vi "DAQAI.vi"(2 "rate":dbl=1000.0, 3 "number of samples":i32=1000, 4 "timeout (s)":dbl=10.0 format="%0.2f", 5 "error in":errorcluster, 7 "stop (F)":bool, 10 "device name":tag="Dev1") -> (14 "task out":refnum<k21>, 15 "data":dynamicdata(graph), 18 "stopped":bool, 19 "error out":errorcluster)   [LabVIEW 2018]
doc: "Creates, edits, and runs tasks using NI-DAQmx. Refer to the NI-DAQmx Readme for a complete listing of devices NI-DAQmx supports.\n\nWhen you place this Express VI on the block diagram, the DAQ Assistant launches to create a new task. After you create a task, you can double-click the DAQ Assistant Express VI to edit that task. For continuous measurement or generation, place a while loop around the DAQ Assistant Express VI."
uses:
  <vilib>/DAQmx/read.llb/DAQmx Read.vi
  <vilib>/DAQmx/read.llb/DAQmx Read (Analog 1D Wfm NChan NSamp).vi
  <vilib>/DAQmx/create/channels.llb/DAQmx Create Channel (TEDS-AI-Voltage-Basic).vi
  <vilib>/DAQmx/create/channels.llb/DAQmx Create Channel (AI-Voltage-Basic).vi
  <vilib>/DAQmx/configure/timing.llb/DAQmx Timing (Sample Clock).vi
  <vilib>/DAQmx/miscellaneous.llb/DAQmx Fill In Error Info.vi
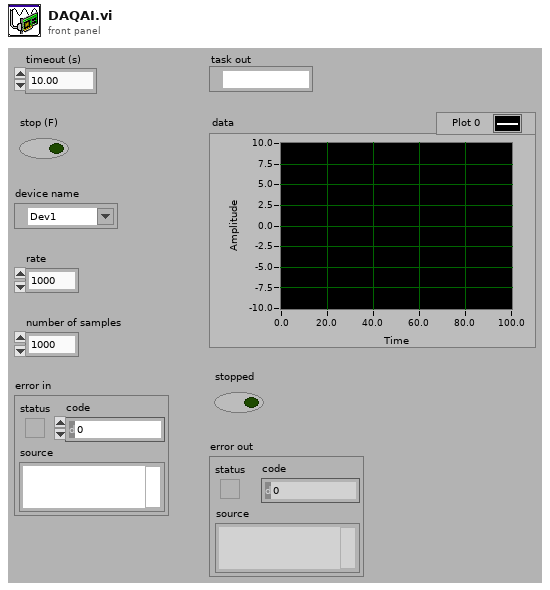
[diagram p1: front panel]
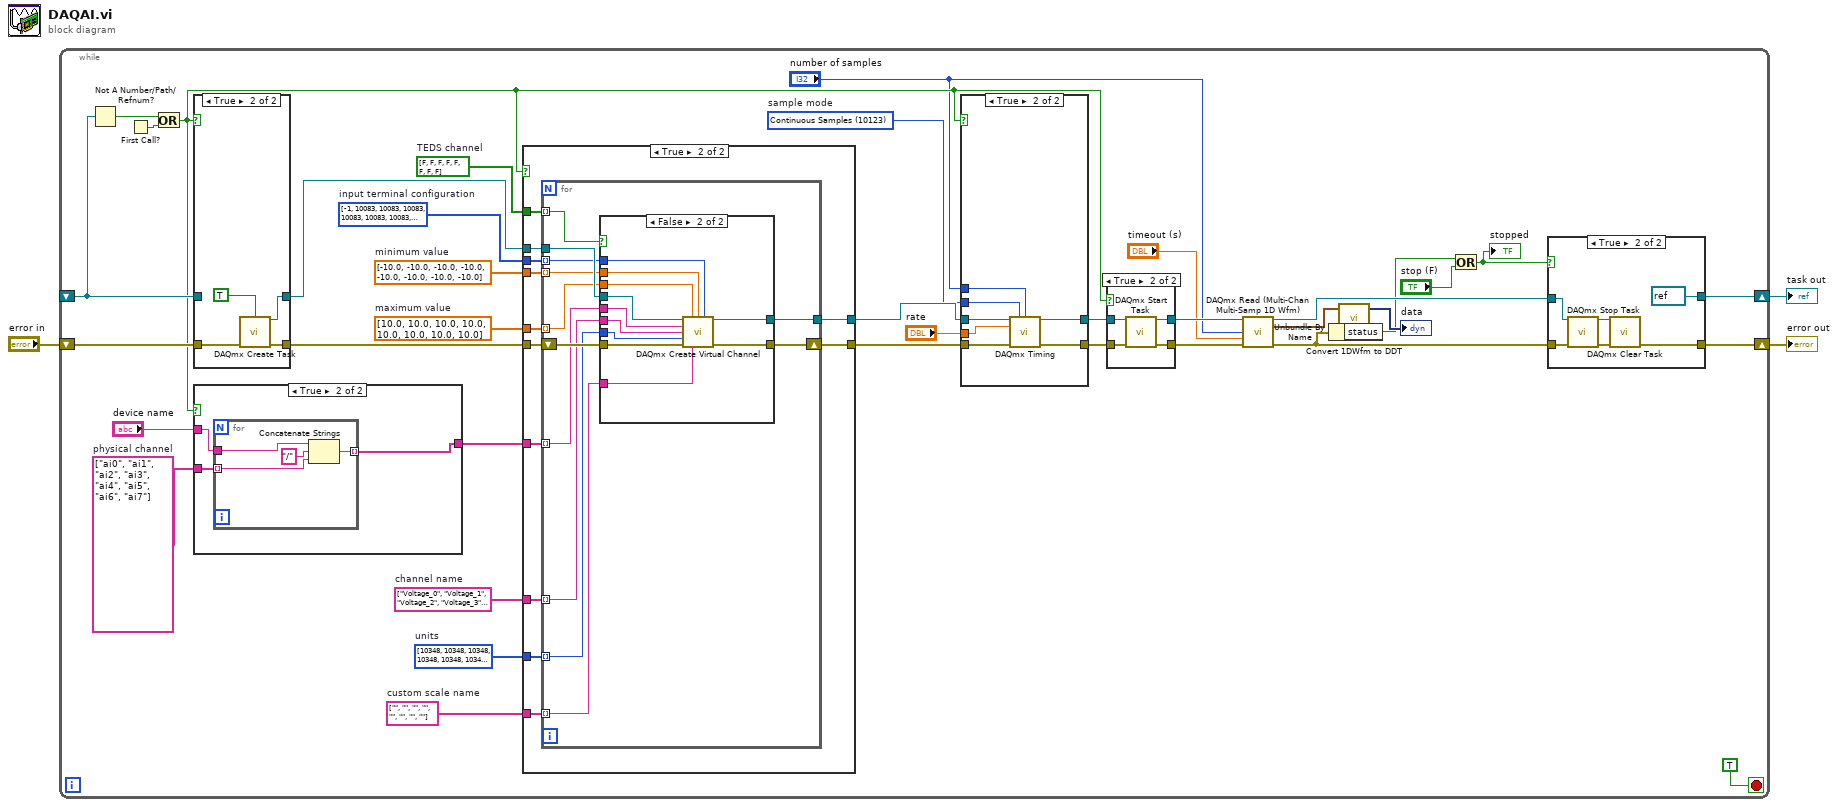
[diagram p0: block diagram]
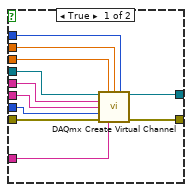
[diagram p6: hidden frame]
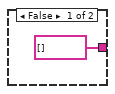
[diagram p7: hidden frame]
diagram:
  n1 = while {
    shift-right: [w10] -> w1
    shift-left: _ -> [w37]
    shift-right: [w8] -> w2
    shift-left: "error in" -> [w38]
    stop <- TRUE stop-if-true
    w20 = 10123 items=["Finite Samples"=10178, "Continuous Samples"=10123, "Hardware Timed Single Point"=12522]  # sample mode
    w24 = bool[] [FALSE, FALSE, FALSE, FALSE, FALSE, FALSE, FALSE, FALSE]  # TEDS channel
    w25 = string[] ["", "", "", "", "", "", "", ""]  # custom scale name
    w26 = i32[] [10348, 10348, 10348, 10348, 10348, 10348, 10348, 10348] items=["Volts"=10348, "From TEDS"=12516, "From Custom Scale"=10065]  # units
    w27 = string[] ["Voltage_0", "Voltage_1", "Voltage_2", "Voltage_3", "Voltage_4", "Voltage_5", "Voltage_6", "Voltage_7"]  # channel name
    w29 = dbl[] [10.0, 10.0, 10.0, 10.0, 10.0, 10.0, 10.0, 10.0]  # maximum value
    w30 = dbl[] [-10.0, -10.0, -10.0, -10.0, -10.0, -10.0, -10.0, -10.0]  # minimum value
    w31 = i32[] [-1, 10083, 10083, 10083, 10083, 10083, 10083, 10083] items=["default"=-1, "RSE"=10083, "NRSE"=10078, "Differential"=10106, "Pseudodifferential"=12529]  # input terminal configuration
    w34 = string[] ["ai0", "ai1", "ai2", "ai3", "ai4", "ai5", "ai6", "ai7"]  # physical channel
    n2 = Not A Number/Path/Refnum?(number/path/refnum=w37) -> (NaN/Path/Refnum?=w36:bool)
    n3 = First Call?() -> (First Call?: T/F=w39:bool)
    n4 = Or(x=w36, y=w39) -> (x .or. y?=w19:bool)
    n5 = case shown="True" w19 {
      tunnel: [w121 w125] -> w33
      tunnel: w37 -> [w121 _]
      tunnel: [w120 w124] -> w32
      tunnel: w38 -> [w120 w122]
      frame False {
      }
      frame True {
        n6 = call <vilib>:"DAQmx Create Task.vi"("auto cleanup"=TRUE, "error in"=w122) -> ("task out"=w125:refnum<k21>, "error out"=w124:errorcluster)  [unwired: 12 in]
      }
    }
    n7 = case shown="True" w19 {
      tunnel: [string[] [] w115] -> w28
      tunnel: "device name" -> [_ w114]
      tunnel: w34 -> [_ w113]
      frame False {
      }
      frame True {
        n8 = for {
          tunnel: [w119] -> w115 mode=indexing
          tunnel: w114 -> [w118]
          tunnel: w113 -> [w116] mode=indexing
          n9 = Concatenate Strings(w118, "/" ("string"), w116) -> (w119:string)
        }
      }
    }
    n10 = case shown="True" w19 {
      tunnel: [w65 w75] -> w23
      tunnel: w33 -> [w65 w77]
      tunnel: [w64 w74] -> w22
      tunnel: w32 -> [w64 w76]
      tunnel: w31 -> [_ w73]
      tunnel: w30 -> [_ w72]
      tunnel: w29 -> [_ w71]
      tunnel: w28 -> [_ w70]
      tunnel: w27 -> [_ w69]
      tunnel: w26 -> [_ w68]
      tunnel: w25 -> [_ w67]
      tunnel: w24 -> [_ w66]
      frame False {
      }
      frame True {
        n11 = for {
          tunnel: w77 -> [w89]
          tunnel: [w87] -> w75
          tunnel: w73 -> [w85] mode=indexing
          tunnel: w72 -> [w84] mode=indexing
          tunnel: w71 -> [w83] mode=indexing
          tunnel: w70 -> [w82] mode=indexing
          tunnel: w69 -> [w81] mode=indexing
          tunnel: w68 -> [w80] mode=indexing
          tunnel: w67 -> [w79] mode=indexing
          shift-right: [w86] -> w74
          shift-left: w76 -> [w88]
          tunnel: w66 -> [w78] mode=indexing
          n12 = case shown="False" w78 {
            tunnel: w89 -> [w100 w111]
            tunnel: w88 -> [w99 w110]
            tunnel: [w98 w109] -> w87
            tunnel: [w97 w108] -> w86
            tunnel: w85 -> [w96 w107]
            tunnel: w84 -> [w95 w106]
            tunnel: w83 -> [w94 w105]
            tunnel: w82 -> [w93 w104]
            tunnel: w81 -> [w92 w103]
            tunnel: w80 -> [w91 w102]
            tunnel: w79 -> [w90 w101]
            frame True {
              n13 = call-poly <vilib>:"DAQmx Create Virtual Channel.vi"("task in"=w100, "maximum value"=w94, "minimum value"=w95, "input terminal configuration"=w96, "physical channels"=w93, "name to assign"=w92, "units"=w91, "error in"=w99, "custom scale name"=w90) -> ("task out"=w98:refnum<k21>, "error out"=w97:errorcluster)  [unwired: 5 in]
            }
            frame False {
              n14 = call-poly <vilib>:"DAQmx Create Virtual Channel.vi"("task in"=w111, "maximum value"=w105, "minimum value"=w106, "input terminal configuration"=w107, "physical channels"=w104, "name to assign"=w103, "units"=w102, "error in"=w110, "custom scale name"=w101) -> ("task out"=w109:refnum<k21>, "error out"=w108:errorcluster)  [unwired: 5 in]
            }
          }
        }
      }
    }
    n15 = case shown="True" w19 {
      tunnel: [w56 w58] -> w18
      tunnel: w23 -> [w56 w61]
      tunnel: [w55 w57] -> w17
      tunnel: w22 -> [w55 w59]
      tunnel: "number of samples" -> [_ w63]
      tunnel: w20 -> [_ w62]
      tunnel: "rate" -> [_ w60]
      frame False {
      }
      frame True {
        n16 = call-poly <vilib>:"DAQmx Timing.vi"("task/channels in"=w61, "sample mode"=w62, "samples per channel"=w63, "rate"=w60, "error in"=w59) -> ("task out"=w58:refnum<k21>, "error out"=w57:errorcluster)  [unwired: 9 in]
      }
    }
    n17 = case shown="True" w19 {
      tunnel: [w50 w53] -> w16
      tunnel: w18 -> [w50 w54]
      tunnel: [w49 w51] -> w15
      tunnel: w17 -> [w49 w52]
      frame False {
      }
      frame True {
        n18 = call <vilib>:"DAQmx Start Task.vi"("task/channels in"=w54, "error in"=w52) -> ("task out"=w53:refnum<k21>, "error out"=w51:errorcluster)  [unwired: 12 in]
      }
    }
    n19 = call-poly "DAQmx Read (Multi-Chan Multi-Samp 1D Wfm).vi"("task/channels in"=w16, "number of samples per channel"="number of samples", "timeout"="timeout (s)", "error in"=w15) -> ("task out"=w9:refnum<k21>, "data"=w13:waveform(dbl)[], "error out"=w7:errorcluster)  [unwired: 9 in]
    n20 = Unbundle By Name(w7) -> ("status"=w6:bool)
    n21 = call <vilib>:"Convert 1DWfm to DDT.vi"("Array of Waveforms"=w13) -> ("Dynamic Data Type"=→"data":dynamicdata)  [unwired: 3 in]
    n22 = Or(x=w6, y="stop (F)") -> (x .or. y?=w4:bool)
    "stopped" <- w4
    n23 = case shown="True" w4 {
      tunnel: [w42 refnum<k21> refnum ("task in")] -> w10
      tunnel: w9 -> [w42 w48]
      tunnel: [w41 w45] -> w8
      tunnel: w7 -> [w41 w47]
      frame False {
      }
      frame True {
        n24 = call <vilib>:"DAQmx Stop Task.vi"("task/channels in"=w48, "error in"=w47) -> ("task out"=w44:refnum<k21>, "error out"=w46:errorcluster)  [unwired: 12 in]
        n25 = call <vilib>:"DAQmx Clear Task.vi"("task in"=w44, "error in"=w46) -> ("error out"=w45:errorcluster)  [unwired: 13 in]
      }
    }
  }
  "error out" <- w2
  "task out" <- w1
